vi "WPI_CAN_Send.vi"(6 "Period (ms)":i32, 8 "error in (no error)":errorcluster, 9 "Data":u8[](array[numeric]), 10 "Message ID":u32 format="%.0x") -> (0 "error out":errorcluster)   [LabVIEW 2017]
doc: "This is the low-level CAN transmit VI. It may be used to communicate with generic CAN devices on the CAN bus.\n\nThis interface currently only supports sending Extended Frames."
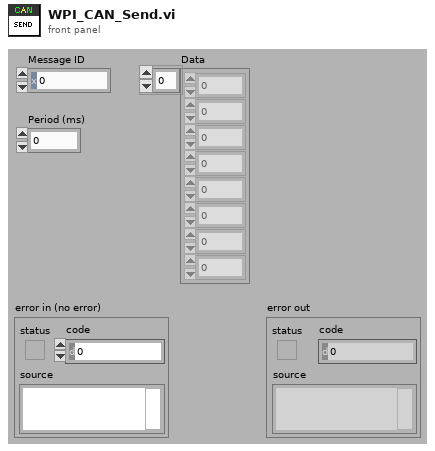
[diagram p1: front panel]
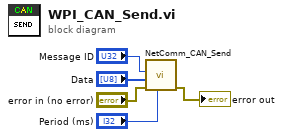
[diagram p0: block diagram]
diagram:
  n1 = call <vilib>:"NetComm_CAN_Send.vi"("Period (ms)"="Period (ms)", "error in (no error)"="error in (no error)", "Data"="Data", "Message ID"="Message ID") -> ("error out"=→"error out":errorcluster)  [unwired: 7 out]
